vi "TestSetLanguage(byVI).vi"(8 "error in (no error)":errorcluster) -> (0 "error out":errorcluster)   [LabVIEW 2017]
uses:
  <vilib>/addons/_JKI Toolkits/Caraya/classes/Test/Test.lvclass
  src/API/JKI Simple Localization.lvlib
  <vilib>/addons/_JKI Toolkits/Caraya/classes/Assert/Assert.lvclass
panel:
  # "See block diagram for unit tests of Set Language (By VI).vi"
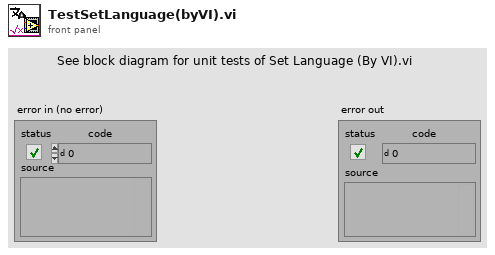
[diagram p1: front panel]
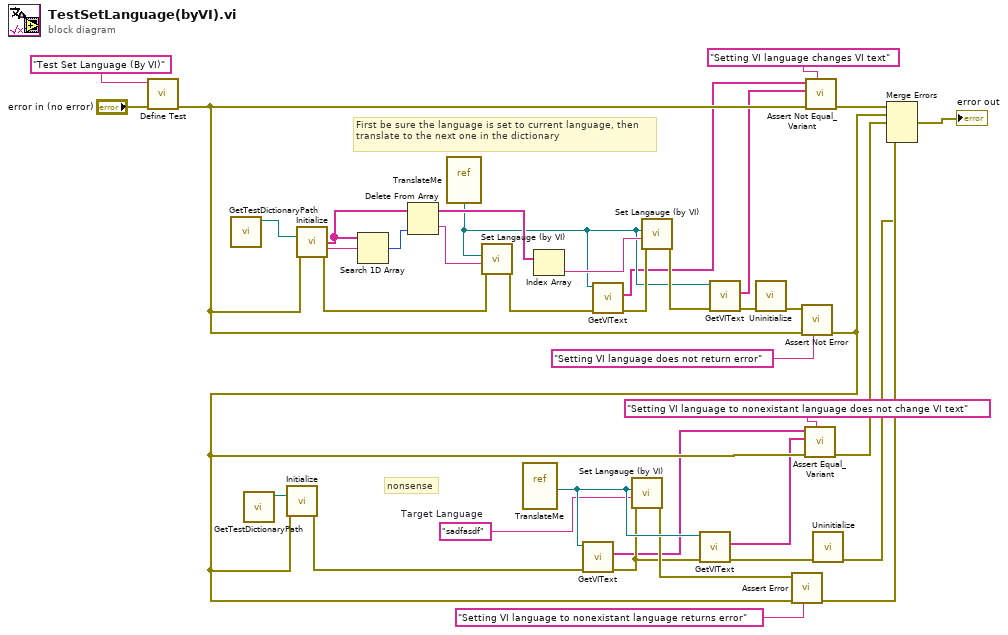
[diagram p0: block diagram]
diagram:
  w24 = "sadfasdf"  # Target Language
  # "nonsense"
  # "First be sure the language is set to current language, then translate to the next one in the dictionary"
  n1 = call <vilib>:"Define Test.vi"("error in (no error)"="error in (no error)", "Label (VI Title)"="Test Set Language (By VI)") -> ("error out"=w21:errorcluster)  [unwired: 9 in]
  n2 = call "GetTestDictionaryPath.vi"() -> ("Test Dictionary Path"=w36:path)  [unwired: 11 in]
  n3 = call "GetTestDictionaryPath.vi"() -> ("Test Dictionary Path"=w23:path)  [unwired: 11 in]
  n4 = call "Initialize.vi"("Dictionary File Path"=w36, "error in"=w21) -> ("Languages"=w30:string[], "Current Language"=w15:string, "error out"=w12:errorcluster)  [unwired: 10 in, 1 out]
  n5 = Search 1D Array(1D array=w30, element=w15) -> (index of element=w31:i32)  [unwired: 1 in]
  n6 = Delete From Array(array=w30, index=w31) -> (deleted portion=w13:string, array with subset deleted=w17:string[])  [unwired: 1 in]
  n7 = vi-ref "TranslateMe.vi"() -> (w14:refnum<vi>)
  n8 = call "Set Langauge (by VI).vi"("error in"=w12, "Target Language"=w13, "VI Ref"=w14) -> ("error out"=w11:errorcluster)  [unwired: 8 in]
  n9 = vi-ref "TranslateMe.vi"() -> (w26:refnum<vi>)
  n10 = Index Array(array=w17) -> (element=w16:string)  [unwired: 1 in]
  n11 = call "GetVIText.vi"("error in (no error)"=w11, "VI"=w14) -> ("error out"=w29:errorcluster, "Control Text"=w4:string[])  [unwired: 6 in, 2 out]
  n12 = call "Set Langauge (by VI).vi"("error in"=w29, "Target Language"=w16, "VI Ref"=w14) -> ("error out"=w28:errorcluster)  [unwired: 8 in]
  n13 = call "GetVIText.vi"("error in (no error)"=w28, "VI"=w14) -> ("error out"=w27:errorcluster, "Control Text"=w3:string[])  [unwired: 6 in, 2 out]
  n14 = call "Uninitialize.vi"("error in"=w27) -> ("error out"=w6:errorcluster)  [unwired: 10 in]
  n15 = call <vilib>:"Assert Not Error.vi"("Label"="Setting VI language does not return error", "error in (no error)"=w21, "Not Error?"=w6) -> ("error out"=w20:errorcluster)  [unwired: 8 in]
  n16 = call "Initialize.vi"("Dictionary File Path"=w23, "error in"=w20) -> ("error out"=w25:errorcluster)  [unwired: 10 in, 3 out]
  n17 = call "GetVIText.vi"("error in (no error)"=w25, "VI"=w26) -> ("error out"=w9:errorcluster, "Control Text"=w2:string[])  [unwired: 6 in, 2 out]
  n18 = call "Set Langauge (by VI).vi"("error in"=w9, "Target Language"=w24, "VI Ref"=w26) -> ("error out"=w10:errorcluster)  [unwired: 8 in]
  n19 = call "GetVIText.vi"("error in (no error)"=w9, "VI"=w26) -> ("error out"=w8:errorcluster, "Control Text"=w1:string[])  [unwired: 6 in, 2 out]
  n20 = call <vilib>:"Assert Error.vi"("Label"="Setting VI language to nonexistant language returns error", "error in (no error)"=w20, "Error?"=w10) -> ("error out"=w7:errorcluster)  [unwired: 8 in]
  n21 = call <vilib>:"Assert Equal_Variant.vi"("Label"="Setting VI language to nonexistant language does not change VI text", "error in (no error)"=w20, "Y"=w1, "X"=w2) -> ("error out"=w18:errorcluster)  [unwired: 7 in]
  n22 = call <vilib>:"Assert Not Equal_Variant.vi"("Label"="Setting VI language changes VI text", "error in (no error)"=w21, "Y"=w3, "X"=w4) -> ("error out"=w34:errorcluster)  [unwired: 7 in]
  n23 = call "Uninitialize.vi"("error in"=w8) -> ("error out"=w5:errorcluster)  [unwired: 10 in]
  n24 = Merge Errors(w34, w20, w18, w5, w7) -> (→"error out":errorcluster)
